vi "Get Channel Status.vi"(1 "Channel":i32=1) -> (0 "body":string)   [LabVIEW 2020]
uses:
  Laser Parameters.vi
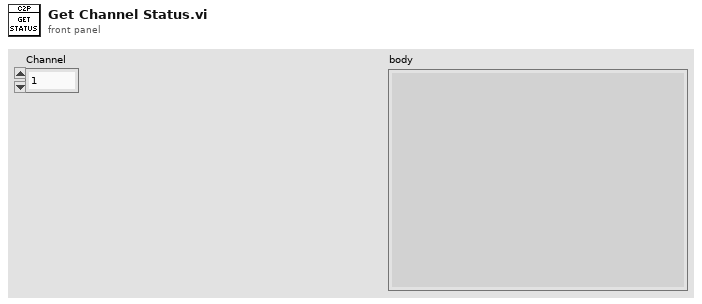
[diagram p1: front panel]
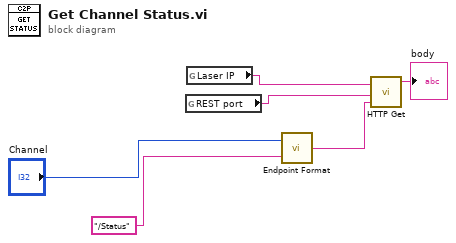
[diagram p0: block diagram]
diagram:
  n1 = global read "Laser Parameters.vi" "REST port"() -> (w5:string)
  n2 = global read "Laser Parameters.vi" "Laser IP"() -> (w6:string)
  n3 = call "Endpoint Format.vi"("Endpoint"="/Status", "Channel"="Channel") -> ("Endpoint URL"=w2:string)
  n4 = call "HTTP Get.vi"("Endpoint"=w2, "Port"=w5, "IP Address"=w6) -> ("body"=→"body":string)  [unwired: 1 in, 1 out]
